vi "Live window-Event handler-Intensity.vi"(7 "Which image display?":T1, 9 "NewVal":cluster{i16, i16}, 11 "OldVal":cluster{i16, i16}) -> ()   [LabVIEW 2013]
uses:
  Typedefs/Left-Right enum.ctl
panel:
  out "error out":errorcluster
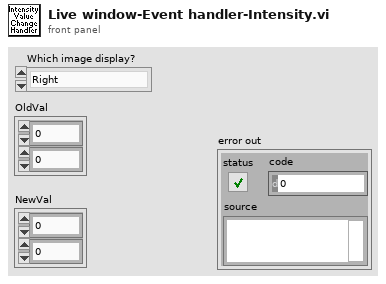
[diagram p1: front panel]
types:
  T1 = typedef "Left-Right enum.ctl" = enum16{"Right", "Left"}
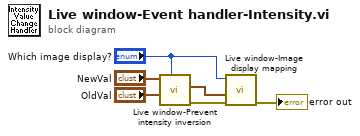
[diagram p0: block diagram]
diagram:
  n1 = call "Live window-Prevent intensity inversion.vi"("Which image display?"="Which image display?", "Old value"="OldVal", "New value"="NewVal") -> ("error out"=w6:errorcluster, "Output setting"=w2:cluster{i16, i16})  [unwired: 7 in]
  n2 = call "Live window-Image display mapping.vi"("error in (no error)"=w6, "Intensity sliders"=w2, "Which image display?"="Which image display?") -> ("error out"=→"error out":errorcluster)  [unwired: 8 in]
